vi "Create Resources.vi"(10 "m_axis_tdata":T1, 11 "m_axis_tvalid":refnum<k21>) -> (3 "niInstr AXI4-Stream Reader FXP64x2 v1 FPGA out":refnum<class "niInstr AXI4-Stream Reader FXP64x2 v1 FPGA.lvclass">)   [LabVIEW 2015, in "niInstr AXI4-Stream Reader FXP64x2 v1 FPGA.lvclass"]
doc: "Creates a new FPGA resource of the selected type.\n\n<b>Do not place this VI into a case structure or it will not compile correctly!</b>\n\n<B>Input Parameters</B>\n\n<B>m_axis_tdata</B> is the resource to use as TDATA.\n\n<B>m_axis_tdata.m_axis_tdata_0</B> is the resource to use for the first portion of TDATA.\n\n<B>m_axis_tdata.m_axis_tdata_1</B> is the resource to use for the second portion of TDATA.\n\n<B>m_axis_tvalid</B> is the resource to use as TVALID.\n\n<B>Output Parameters</B>\n\n<B>niInstr AXI4-Stream Reader FXP64x2 v1 FPGA out</B> passes a reference to the AXI4-Stream Reader to the next VI."
uses:
  <instrlib>/_niInstr/CLIP Adapters/v1/FPGA/AXI4-Stream/Reader FXP64x2/niInstr AXI4-Stream Reader FXP64x2 v1 FPGA.lvclass
  <instrlib>/_niInstr/CLIP Adapters/v1/FPGA/AXI4-Stream/Reader FXP64x2/Public/m_axis_tdata.ctl
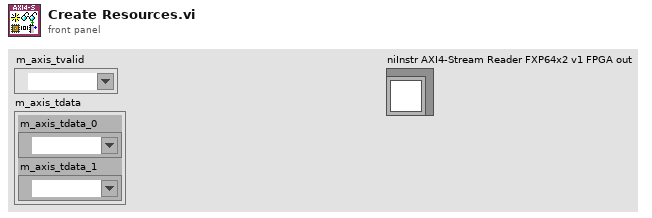
[diagram p1: front panel]
types:
  T1 = typedef "niInstr AXI4-Stream Reader FXP64x2 v1 FPGA.lvclass/m_axis_tdata.ctl" = cluster{"m_axis_tdata_0":refnum<k21>, "m_axis_tdata_1":refnum<k21>}
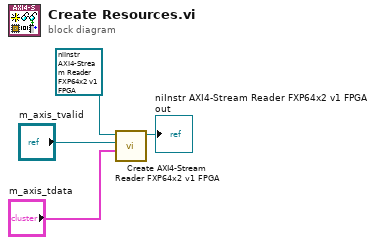
[diagram p0: block diagram]
diagram:
  n1 = call <instrlib>:"Create AXI4-Stream Reader FXP64x2 v1 FPGA.vi"("tdata resources"="m_axis_tdata", "tvalid"="m_axis_tvalid", "niInstr AXI4-Stream Reader FXP64x2 v1 FPGA in"=refnum<class "niInstr AXI4-Stream Reader FXP64x2 v1 FPGA.lvclass"> refnum ("Reader in")) -> ("niInstr AXI4-Stream Reader FXP64x2 v1 FPGA out"=→"niInstr AXI4-Stream Reader FXP64x2 v1 FPGA out":refnum<class "niInstr AXI4-Stream Reader FXP64x2 v1 FPGA.lvclass">)  [unwired: 8 in]
